vi "Find Next Position of T.vi"(0 "Current Position of T":cdb, 1 "Current Position of H":cdb) -> (2 "Next Position of T":cdb)   [LabVIEW 2020, in "AoC 2022.lvlib"]
uses:
  AoC 2022.lvlib
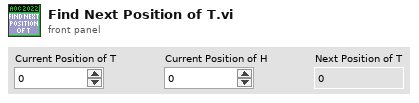
[diagram p1: front panel]
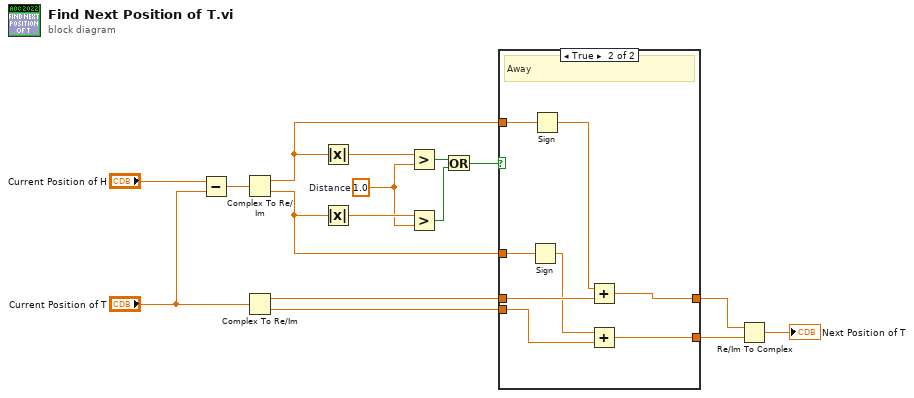
[diagram p0: block diagram]
diagram:
  w8 = 1.0  # Distance
  n1 = Subtract(x="Current Position of H", y="Current Position of T") -> (x-y=w13:cdb)
  n2 = Complex To Re/Im(x + iy=w13) -> (x=w12:dbl, y=w11:dbl)
  n3 = Complex To Re/Im(x + iy="Current Position of T") -> (x=w7:dbl, y=w6:dbl)
  n4 = Absolute Value(x=w12) -> (abs(x)=w10:dbl)
  n5 = Absolute Value(x=w11) -> (abs(x)=w9:dbl)
  n6 = Greater?(x=w10, y=w8) -> (0:w3:bool)
  n7 = Greater?(x=w9, y=w8) -> (0:w2:bool)
  n8 = Or(x=w3, y=w2) -> (x .or. y?=w1:bool)
  n9 = case shown="True" w1 {
    tunnel: w12 -> [_ w26]
    tunnel: w11 -> [_ w25]
    tunnel: w7 -> [w18 w24]
    tunnel: w6 -> [w17 w21]
    tunnel: [w18 w22] -> w5
    tunnel: [w17 w19] -> w4
    frame False {
      # "Touching"
    }
    frame True {
      # "Away"
      n10 = Sign(1:w25) -> (0:w20:dbl)
      n11 = Sign(1:w26) -> (0:w23:dbl)
      n12 = Add(x=w23, y=w24) -> (x+y=w22:dbl)
      n13 = Add(x=w20, y=w21) -> (x+y=w19:dbl)
    }
  }
  n14 = Re/Im To Complex(1:w4, 2:w5) -> (0:→"Next Position of T":cdb)
